vi "Aux TE Controllers Runtime (2).vi"(8 "Error In":errorcluster, 9 "TE Serial Ports In":T4[](array[typedef]) {"XOFF Char" format="%.0x"; "XON Char" format="%.0x"; "flow control" items=["None"=0, "XON/XOFF"=1, "RTS/CTS"=2, "DTR/DSR"=4]; "stop bits" items=["1.0"=10, "1.5"=15, "2.0"=20]; "data bits" min=5 max=8 step=1; "baud rate" items=["75"=75, "110"=110, "134"=134, "150"=150, "300"=300, "600"=600, "1200"=1200, "1800"=1800, "2400"=2400, "4800"=4800, "7200"=7200, "9600"=9600, "14400"=14400, "19200"=19200, "28800"=28800, "38400"=38400, "56000"=56000, "57600"=57600, "115200"=115200, "128000"=128000, "230400"=230400]; "termination char" format="%.0x"}, 10 "CmdsToWrite":string[](array[string]), 11 "Refs":T1 {"Current Settings"."Pump" items=["Pump 0", "Pump 1", "Pump 2", "Pump 3", "Pump 4", "Pump 5"]; "Current Settings"."Chart X axis Timescale" min=20 max=180 step=1; "Current Settings"."RunTime Mode Settings"."Exp. Gas Tank" items=["0.07", "0.031", "0.877", "1.863", "3.881", "5.790", "7.688", "6.000"]; "Current Settings"."RunTime Mode Settings"."Insp. Gas Tank" items=["0.07", "0.031", "0.877", "1.863", "3.881", "5.790", "7.688", "6.000"]; "Current Settings"."RunTime Mode Settings"."I:E Ratio" max=30 scale=0.0..7.0; "Current Settings"."RunTime Mode Settings"."Resp Rate Brpm" min=0 max=30 format="%.2f"; "Current Settings"."TE#2 Configuration"."Serial Port"."XOFF Char" format="%.0x"; "Current Settings"."TE#2 Configuration"."Serial Port"."XON Char" format="%.0x"; "Current Settings"."TE#2 Configuration"."Serial Port"."flow control" items=["None"=0, "XON/XOFF"=1, "RTS/CTS"=2, "DTR/DSR"=4]; "Current Settings"."TE#2 Configuration"."Serial Port"."stop bits" items=["1.0"=10, "1.5"=15, "2.0"=20]; "Current Settings"."TE#2 Configuration"."Serial Port"."data bits" min=5 max=8 step=1; "Current Settings"."TE#2 Configuration"."Serial Port"."baud rate" items=["75"=75, "110"=110, "134"=134, "150"=150, "300"=300, "600"=600, "1200"=1200, "1800"=1800, "2400"=2400, "4800"=4800, "7200"=7200, "9600"=9600, "14400"=14400, "19200"=19200, "28800"=28800, "38400"=38400, "56000"=56000, "57600"=57600, "115200"=115200, "128000"=128000, "230400"=230400]; "Current Settings"."TE#2 Configuration"."Serial Port"."termination char" format="%.0x"; "Current Settings"."TE#1 Configuration"."Serial Port"."XOFF Char" format="%.0x"; "Current Settings"."TE#1 Configuration"."Serial Port"."XON Char" format="%.0x"; "Current Settings"."TE#1 Configuration"."Serial Port"."flow control" items=["None"=0, "XON/XOFF"=1, "RTS/CTS"=2, "DTR/DSR"=4]; "Current Settings"."TE#1 Configuration"."Serial Port"."stop bits" items=["1.0"=10, "1.5"=15, "2.0"=20]; "Current Settings"."TE#1 Configuration"."Serial Port"."data bits" min=5 max=8 step=1; "Current Settings"."TE#1 Configuration"."Serial Port"."baud rate" items=["75"=75, "110"=110, "134"=134, "150"=150, "300"=300, "600"=600, "1200"=1200, "1800"=1800, "2400"=2400, "4800"=4800, "7200"=7200, "9600"=9600, "14400"=14400, "19200"=19200, "28800"=28800, "38400"=38400, "56000"=56000, "57600"=57600, "115200"=115200, "128000"=128000, "230400"=230400]; "Current Settings"."TE#1 Configuration"."Serial Port"."termination char" format="%.0x"; "Current Settings"."Capnometer Configuration"."Device" items=["None", "TidalWave", "LoFlow / Canary", "Capnogard"]; "Current Settings"."Capnometer Configuration"."Serial Port"."XOFF Char" format="%.0x"; "Current Settings"."Capnometer Configuration"."Serial Port"."XON Char" format="%.0x"; "Current Settings"."Capnometer Configuration"."Serial Port"."flow control" items=["None"=0, "XON/XOFF"=1, "RTS/CTS"=2, "DTR/DSR"=4]; "Current Settings"."Capnometer Configuration"."Serial Port"."stop bits" items=["1.0"=10, "1.5"=15, "2.0"=20]; "Current Settings"."Capnometer Configuration"."Serial Port"."data bits" min=5 max=8 step=1; "Current Settings"."Capnometer Configuration"."Serial Port"."baud rate" items=["75"=75, "110"=110, "134"=134, "150"=150, "300"=300, "600"=600, "1200"=1200, "1800"=1800, "2400"=2400, "4800"=4800, "7200"=7200, "9600"=9600, "14400"=14400, "19200"=19200, "28800"=28800, "38400"=38400, "56000"=56000, "57600"=57600, "115200"=115200, "128000"=128000, "230400"=230400]; "Current Settings"."Capnometer Configuration"."Serial Port"."termination char" format="%.0x"; "Current Settings"."DAQx Settings"."Analog Output Settings (Volts)" format="%#.3g"; "Current Settings"."DAQx Settings"."Duty Cycle" min=10.0 max=90.0 format="%.1g"; "Current Settings"."DAQx Settings"."Frequency" min=20.0 max=200.0; "Current Settings"."DataLogging Settings"."Data File Duration (Minutes)" min=2 max=200 format="%#.2g"; "Current Settings"."Calibration Settings"."Tolerance #2" min=2 max=4096; "Current Settings"."Calibration Settings"."Cal. Average" min=2 max=4096; "Current Settings"."Test Settings"."Test Sensor ID" items=["(select)", "RB", "YC", "", "Other"]}) -> (0 "Error Out":errorcluster, 1 "Read Array":string[][](array[string]), 2 "ReadData":sgl[][](array[numeric]) format="%.2g", 3 "TE Serial Ports Out":T4[](array[typedef]) {"XOFF Char" format="%.0x"; "XON Char" format="%.0x"; "flow control" items=["None"=0, "XON/XOFF"=1, "RTS/CTS"=2, "DTR/DSR"=4]; "stop bits" items=["1.0"=10, "1.5"=15, "2.0"=20]; "data bits" min=5 max=8 step=1; "baud rate" items=["75"=75, "110"=110, "134"=134, "150"=150, "300"=300, "600"=600, "1200"=1200, "1800"=1800, "2400"=2400, "4800"=4800, "7200"=7200, "9600"=9600, "14400"=14400, "19200"=19200, "28800"=28800, "38400"=38400, "56000"=56000, "57600"=57600, "115200"=115200, "128000"=128000, "230400"=230400]; "termination char" format="%.0x"}, 4 "TE Bytes Read":i16[][](array[numeric]), 5 "Set Point Good":bool, 6 "TE Data":sgl[][](array[numeric]), 7 "Set Point Disabled":bool)   [LabVIEW 2015]
uses:
  Controls/Serial Visa Control.ctl
  Controls/DAQ Needed.ctl
  Controls/Processed Variables.ctl
  Controls/AirPump Controls.ctl
  Controls/IE Ratio knob.ctl
  Controls/UI Settings.ctl
  Controls/Aux CO2 Control.ctl
  Controls/Aux CO2 Selector.ctl
  Controls/Aux TE Control.ctl
  Controls/Queues And Others.ctl
  Controls/SerialPortControl.ctl
  Miscellaneous/Globals.vi
panel:
  out "after substring":string
  out "appended array":string[][](array[string])
  out "subarray":dbl[](array[numeric])
  out "size(s)":i32[](array[numeric])
  # "Note: Setting Brpm to zero will\ndisable Insp / Exp digital output."
  # "mmHg"
  # "pts"
  # "tolerance"
  # "AN5 (Temp 1)"
  # "AN6 (Temp 2)"
  # "AN7 (Temp 3)"
  # "AN8 (T FET)"
  # "AN0 (T POT)"
  # "Tref (Set Pt))"
  # "(Spare)"
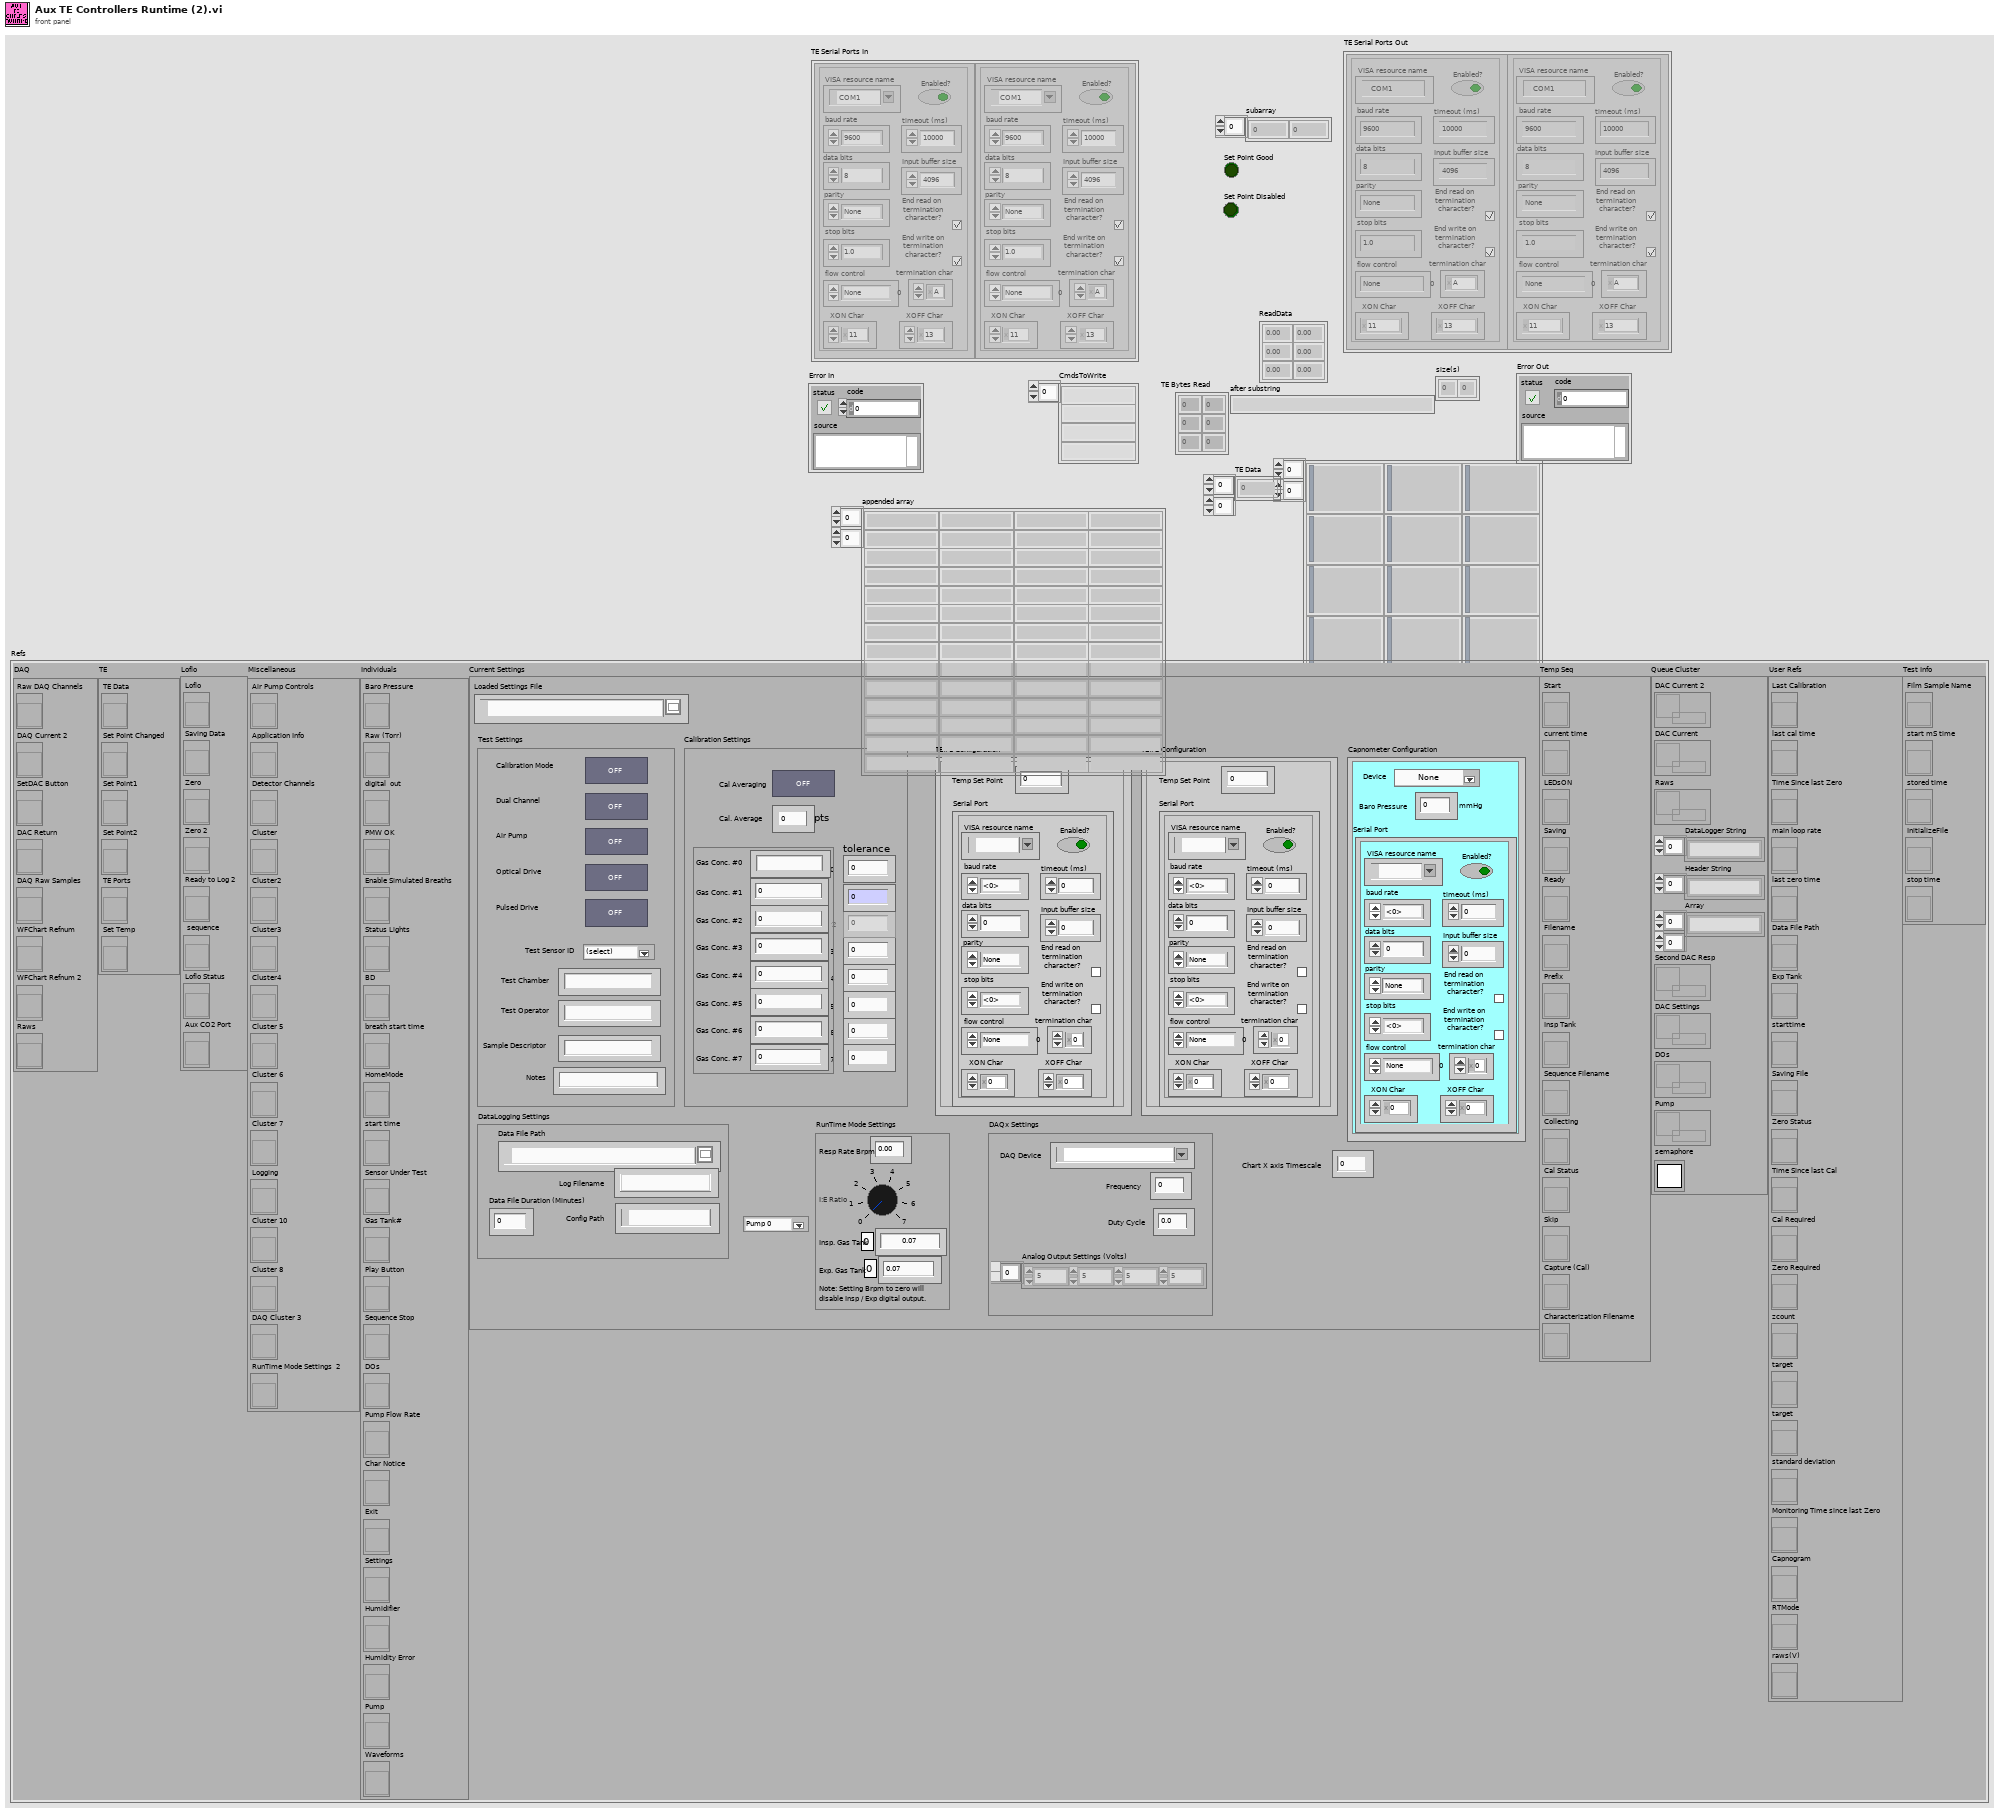
[diagram p1: front panel]
types:
  T1 = typedef "DAQ Needed.ctl" = cluster{"DAQ":cluster{"Raw DAQ Channels":refnum<vi>, "DAQ Current 2":refnum<vi>, "SetDAC Button":refnum<vi>, "DAC Return":refnum<vi>, "DAQ Raw Samples":refnum<vi>, "WFChart Refnum":refnum<vi>, "WFChart Refnum 2":refnum<vi>, "Raws":refnum<vi>}, "TE":cluster{"TE Data":refnum<vi>, "Set Point Changed":refnum<vi>, "Set Point1":refnum<vi>, "Set Point2":refnum<vi>, "TE Ports":refnum<vi>, "Set Temp":refnum<vi>}, "Loflo":cluster{"Loflo":refnum<vi>, "Saving Data":refnum<vi>, "Zero":refnum<vi>, "Zero 2":refnum<vi>, "Ready to Log 2":refnum<vi>, " sequence":refnum<vi>, "Loflo Status ":refnum<vi>, "Aux CO2 Port":refnum<vi>}, "Miscellaneous":cluster{"Air Pump Controls":refnum<vi>, "Application Info":refnum<vi>, "Detector Channels ":refnum<vi>, "Cluster":refnum<vi>, "Cluster2":refnum<vi>, "Cluster3":refnum<vi>, "Cluster4":refnum<vi>, "Cluster 5":refnum<vi>, "Cluster 6":refnum<vi>, "Cluster 7":refnum<vi>, "Logging":refnum<vi>, "Cluster 10":refnum<vi>, "Cluster 8":refnum<vi>, "DAQ Cluster 3":refnum<vi>, "RunTime Mode Settings  2":refnum<vi>}, "Individuals":cluster{"Baro Pressure":refnum<vi>, "Raw (Torr)":refnum<vi>, "digital  out":refnum<vi>, "PMW OK":refnum<vi>, "Enable Simulated Breaths":refnum<vi>, "Status Lights":refnum<vi>, "BD":refnum<vi>, "breath start time":refnum<vi>, "HomeMode":refnum<vi>, "start time":refnum<vi>, "Sensor Under Test":refnum<vi>, "Gas Tank#":refnum<vi>, "Play Button":refnum<vi>, "Sequence Stop":refnum<vi>, "DOs":refnum<vi>, "Pump Flow Rate":refnum<vi>, "Char Notice":refnum<vi>, "Exit":refnum<vi>, "Settings":refnum<vi>, "Humidifier":refnum<vi>, "Humidity Error":refnum<vi>, "Pump":refnum<vi>, "Waveforms":refnum<vi>}, "Current Settings":T2, "Temp Seq":cluster{"Start":refnum<vi>, "current time":refnum<vi>, "LEDsON":refnum<vi>, "Saving":refnum<vi>, "Ready":refnum<vi>, "Filename":refnum<vi>, "Prefix":refnum<vi>, "Insp Tank":refnum<vi>, "Sequence Filename":refnum<vi>, "Collecting":refnum<vi>, "Cal Status":refnum<vi>, "Skip":refnum<vi>, "Capture (Cal)":refnum<vi>, "Characterization Filename":refnum<vi>}, "Queue Cluster":T7, "User Refs":cluster{"Last Calibration":refnum<vi>, "last cal time":refnum<vi>, "Time Since last Zero":refnum<vi>, "main loop rate":refnum<vi>, "last zero time":refnum<vi>, "Data File Path":refnum<vi>, "Exp Tank":refnum<vi>, "starttime":refnum<vi>, "Saving File":refnum<vi>, "Zero Status":refnum<vi>, "Time Since last Cal":refnum<vi>, "Cal Required":refnum<vi>, "Zero Required":refnum<vi>, "zcount":refnum<vi>, "target":refnum<vi>, "target":refnum<vi>, "standard deviation":refnum<vi>, "Monitoring Time since last Zero":refnum<vi>, "Capnogram":refnum<vi>, "RTMode":refnum<vi>, "raws(V)":refnum<vi>}, "Test Info":cluster{"Film Sample Name":refnum<vi>, "start mS time":refnum<vi>, "stored time":refnum<vi>, "InitializeFile":refnum<vi>, "stop time":refnum<vi>}}
  T2 = typedef "UI Settings.ctl" = cluster{"Loaded Settings File":path, "Test Settings":cluster{"Dual Channel":bool, "Air Pump":bool, "Optical Drive":bool, "Pulsed Drive":bool, "Calibration Mode":bool, "Test Sensor ID":u16, "Test Chamber":string, "Test Operator":string, "Sample Descriptor":string, "Notes":string}, "Calibration Settings":cluster{"Cal. Average":u16, "Cal Averaging":bool, "Tolerance #0":sgl, "Tolerance #7":sgl, "Tolerance #6":sgl, "Tolerance #5":sgl, "Tolerance #4":sgl, "Tolerance #3":sgl, "Tolerance #2":sgl, "Tolerance #1":sgl, "Gas Tank Settings":cluster{"Gas Conc. #0":string, "Gas Conc. #1":sgl, "Gas Conc. #2":sgl, "Gas Conc. #3":sgl, "Gas Conc. #4":sgl, "Gas Conc. #5":sgl, "Gas Conc. #6":sgl, "Gas Conc. #7":sgl}}, "DataLogging Settings":cluster{"Data File Path":path, "Data File Duration (Minutes)":sgl, "Log Filename":string, "Config Path":path}, "DAQx Settings":cluster{"DAQ Device":tag, "Frequency":dbl, "Duty Cycle":dbl, "Analog Output Settings (Volts)":sgl[]}, "Capnometer Configuration":T3, "TE#1 Configuration":T6, "TE#2 Configuration":T6, "RunTime Mode Settings ":cluster{"Resp Rate Brpm ":sgl, "I:E Ratio":u8, "Insp. Gas Tank":u16, "Exp. Gas Tank":u16}, "Chart X axis Timescale":u16, "Pump":u16}
  T3 = typedef "Aux CO2 Control.ctl" = cluster{"Serial Port":T4, "Baro Pressure":u32, "Device":T5}
  T4 = typedef "Serial Visa Control.ctl" = cluster{"termination char":u8, "End read on termination character?":bool, "Enabled?":bool, "VISA resource name":refnum<visa-resource-name>, "baud rate":u32, "data bits":u16, "parity":enum16{"None", "Odd", "Even", "Mark", "Space"}, "stop bits":u16, "flow control":u16, "timeout (ms)":u32, "Input buffer size":u32, "End write on termination character?":bool, "XON Char":u8, "XOFF Char":u8}
  T5 = typedef "Aux CO2 Selector.ctl" = u16
  T6 = typedef "Aux TE Control.ctl" = cluster{"Temp Set Point":sgl, "Serial Port":T4}
  T7 = typedef "Queues And Others.ctl" = cluster{"DAC Current 2":refnum<queue>, "DAC Current":refnum<queue>, "Raws":refnum<queue>, "DataLogger String":string[], "Header String":string[], "Array":string[][], "Second DAC Resp":refnum<queue>, "DAC Settings":refnum<queue>, "DOs":refnum<queue>, "Pump":refnum<queue>, "semaphore":T8}
  T8 = typedef "Semaphore RefNum" = refnum<k1>
  T9 = typedef "SerialPortControl.ctl" = enum16{"Initialize", "Write Data", "Read Data", "Close Port"}
  T10 = cluster{"Ref CO2":sgl, "Humidity":sgl, "TE #1":sgl, "TE #2":sgl, " Film `C":dbl, "Bath `C":dbl, " Det. `C":dbl, " Ambient":dbl, " Chamber C ":dbl}
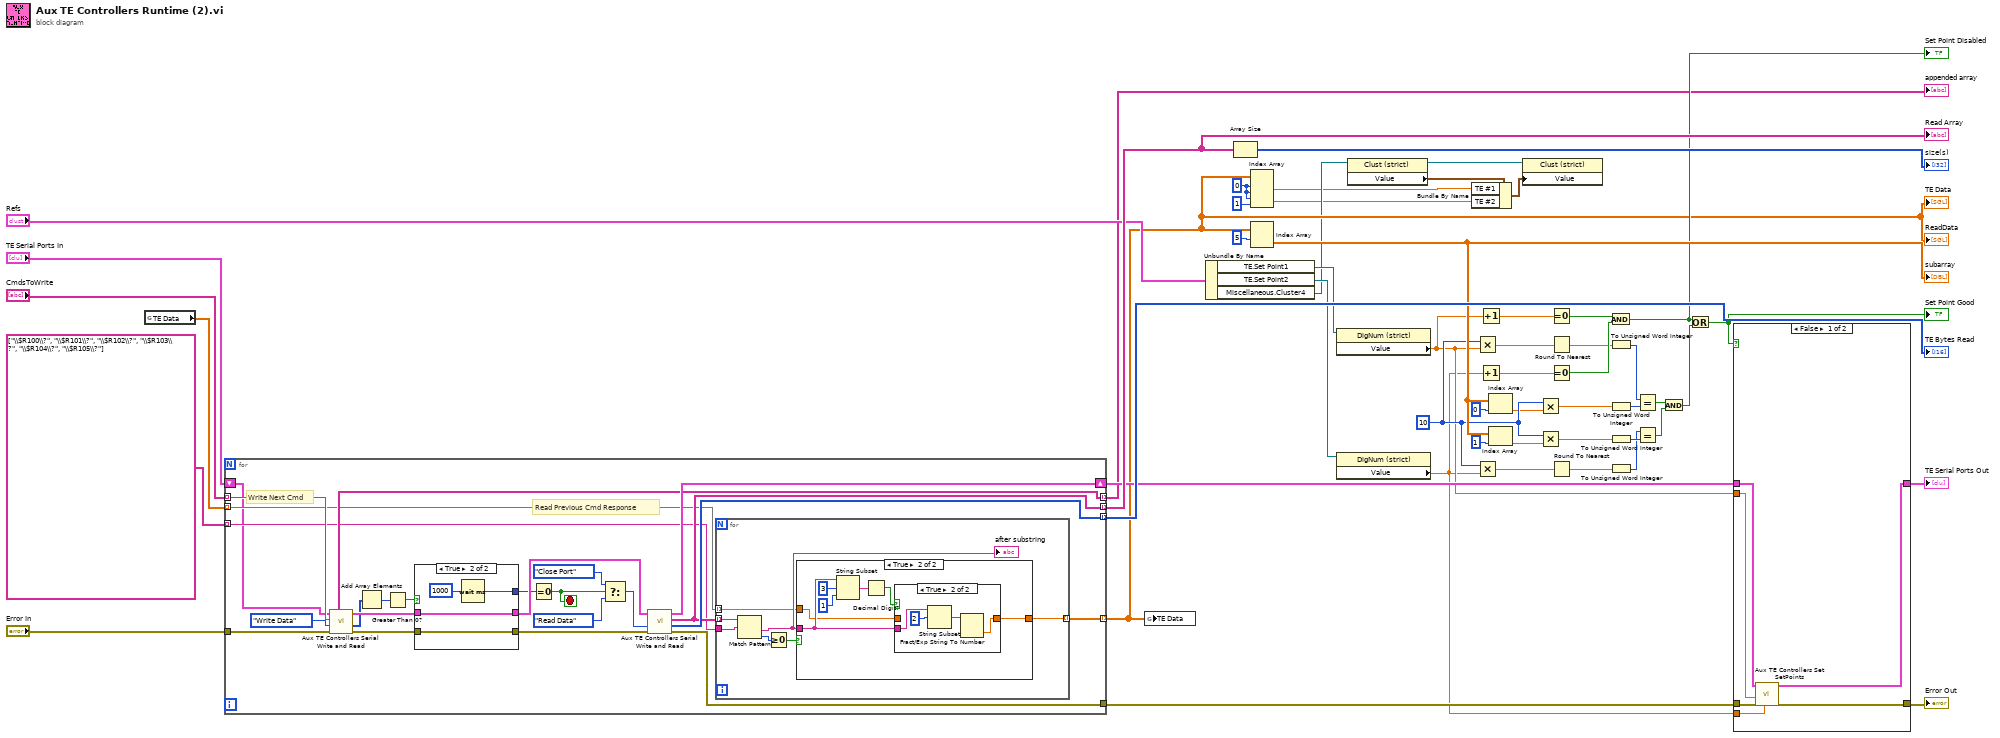
[diagram p0: block diagram]
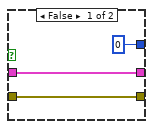
[diagram p5: hidden frame]
diagram:
  w16 = 0 ("index (row)")
  w40 = 10
  n1 = global read "Globals.vi" "TE Data"() -> (w10:sgl[][])
  n2 = for {
    tunnel: [w74] -> w33
    tunnel: "Error In" -> [w76]
    tunnel: [w73] -> w51 mode=indexing
    tunnel: "CmdsToWrite" -> [w58] mode=indexing
    tunnel: [w59] -> w52 mode=indexing
    tunnel: [w57] -> w9 mode=indexing
    tunnel: [w60] -> w11 mode=indexing
    tunnel: string[] ["\\$R100\\?", "\\$R101\\?", "\\$R102\\?", "\\$R103\\?", "\\$R104\\?", "\\$R105\\?"] ("CmdsToWrite") -> [w56] mode=indexing
    tunnel: w10 -> [w55] mode=indexing
    shift-right: [w75] -> w35
    shift-left: "TE Serial Ports In" -> [w54]
    stop <- w61 stop-if-true
    # "Read Previous Cmd Response"
    # "Write Next Cmd"
    n3 = call "Aux TE Controllers Serial Write and Read.vi"("error in"=w76, "Action"=SerialPortControl."Write Data", "string to write"=w58, "TE Controller Serial Ports In"=w54) -> ("Error Out"=w70:errorcluster, "#Bytes R/W"=w66:i16[], "TE Controller Serial Ports Out"=w72:T4[], "appended array"=w60:string[])  [unwired: 1 in, 1 out]
    n4 = Add Array Elements(numeric array=w66) -> (sum=w68:i16)
    n5 = Greater Than 0?(x=w68) -> (x > 0?=w67:bool)
    n6 = case shown="True" w67 {
      tunnel: [w99 w104] -> w71
      tunnel: w72 -> [w99 w104]
      tunnel: [w100 w103] -> w69
      tunnel: w70 -> [w100 w103]
      tunnel: [u32 0 ("millisecond timer value") w101] -> w65
      frame False {
      }
      frame True {
        n7 = Wait (ms)(milliseconds to wait=i16 1000 ("y")) -> (millisecond timer value=w101:u32)
      }
    }
    n8 = Equal To 0?(x=w65) -> (x = 0?=w61:bool)
    n9 = Select(t=SerialPortControl."Close Port" ("Action"), s=w61, f=SerialPortControl."Read Data" ("Action")) -> (s? t:f=w64:T9)
    n10 = call "Aux TE Controllers Serial Write and Read.vi"("error in"=w69, "Action"=w64, "TE Controller Serial Ports In"=w71) -> ("Error Out"=w74:errorcluster, "#Bytes R/W"=w73:i16[], "Data Read"=w59:string[], "TE Controller Serial Ports Out"=w75:T4[])  [unwired: 2 in, 1 out]
    n11 = for {
      tunnel: w59 -> [w84] mode=indexing
      tunnel: w56 -> [w83]
      tunnel: [w81] -> w57 mode=indexing
      tunnel: w55 -> [w80] mode=indexing
      n12 = Match Pattern(string=w84, regular expression=w83) -> (after substring=w82:string, offset past match=w79:i32)  [unwired: 1 in, 2 out]
      "after substring" <- w82
      n13 = Greater Or Equal To 0?(x=w79) -> (x >= 0?=w78:bool)
      n14 = case shown="True" w78 {
        tunnel: w82 -> [_ w87]
        tunnel: [w85 w92] -> w81
        tunnel: w80 -> [w85 w86]
        frame False {
        }
        frame True {
          n15 = String Subset(string=w87, offset (0)=3, length (rest)=1 ("length (rest)")) -> (substring=w89:string)
          n16 = Decimal Digit?(1:w89) -> (0:w88:bool)
          n17 = case shown="True" w88 {
            tunnel: [w93 w97] -> w92
            tunnel: w87 -> [_ w95]
            tunnel: w86 -> [w93 _]
            frame False {
            }
            frame True {
              n18 = String Subset(string=w95, offset (0)=2) -> (substring=w94:string)  [unwired: 1 in]
              n19 = Fract/Exp String To Number(string=w94) -> (number=w97:dbl)  [unwired: 3 in, 1 out]
            }
          }
        }
      }
    }
  }
  "TE Bytes Read" <- w51
  "Read Array" <- w52
  "ReadData" <- w9
  "TE Data" <- w9
  "appended array" <- w11
  n20 = global write "Globals.vi" "TE Data"(w9) -> ()
  n21 = Unbundle By Name("Refs") -> ("TE.Set Point1"=w13:refnum<vi>, "TE.Set Point2"=w12:refnum<vi>, "Miscellaneous.Cluster4"=w6:refnum<vi>)
  n22 = Array Size(array=w52) -> (size(s)=→"size(s)":i32[])
  n23 = Index Array(array=w9, index (row) #1=w16, index (col) #1=w16, index (row) #2=w16, index (col) #2=1 ("disabled index (col)")) -> (element #1=w2:dbl, element #2=w1:dbl)
  n24 = Index Array(array=w9, index (row)=5) -> (element=w45:dbl[])  [unwired: 1 in]
  "subarray" <- w45
  n25 = property class="DigNum (strict)"(reference=w13) -> ("Value"=w18:sgl)  [unwired: 1 in, 2 out]
  n26 = property class="DigNum (strict)"(reference=w12) -> ("Value"=w17:sgl)  [unwired: 1 in, 2 out]
  n27 = property class="Clust (strict)"(reference=w6) -> (reference out=w5:refnum<vi>, "Value"=w4:T10)  [unwired: 1 in, 1 out]
  n28 = Bundle By Name(cluster=w4, "TE #1"=w2, "TE #2"=w1) -> (w3:T10)
  n29 = Multiply(x=w40, y=w18) -> (x*y=w21:sgl)
  n30 = Multiply(x=w40, y=w17) -> (x*y=w23:sgl)
  n31 = Increment(x=w18) -> (x+1=w31:sgl)
  n32 = Increment(x=w17) -> (x+1=w30:sgl)
  n33 = Index Array(array=w45, index=0) -> (element=w39:dbl)
  n34 = Index Array(array=w45, index=1) -> (element=w41:dbl)
  n35 = property class="Clust (strict)"(reference=w5, "Value"=w3) -> ()  [unwired: 1 in, 2 out]
  n36 = Multiply(x=w40, y=w39) -> (x*y=w22:dbl)
  n37 = Multiply(x=w40, y=w41) -> (x*y=w24:dbl)
  n38 = Equal To 0?(x=w31) -> (x = 0?=w28:bool)
  n39 = Round To Nearest(number=w21) -> (nearest integer value=w20:sgl)
  n40 = Equal To 0?(x=w30) -> (x = 0?=w29:bool)
  n41 = Round To Nearest(number=w23) -> (nearest integer value=w19:sgl)
  n42 = And(x=w28, y=w29) -> (x .and. y?=w25:bool)
  "Set Point Disabled" <- w25
  n43 = To Unsigned Word Integer(number=w20) -> (unsigned 16bit integer=w36:u16)
  n44 = To Unsigned Word Integer(number=w22) -> (unsigned 16bit integer=w37:u16)
  n45 = To Unsigned Word Integer(number=w24) -> (unsigned 16bit integer=w42:u16)
  n46 = To Unsigned Word Integer(number=w19) -> (unsigned 16bit integer=w38:u16)
  n47 = Equal?(x=w36, y=w37) -> (x = y?=w43:bool)
  n48 = Equal?(x=w38, y=w42) -> (x = y?=w44:bool)
  n49 = And(x=w43, y=w44) -> (x .and. y?=w27:bool)
  n50 = Or(x=w25, y=w27) -> (x .or. y?=w26:bool)
  "Set Point Good" <- w26
  n51 = case shown="False" w26 {
    tunnel: [w107 w112] -> w34
    tunnel: w35 -> [w110 w112]
    tunnel: [w108 w111] -> w32
    tunnel: w33 -> [w109 w111]
    tunnel: w18 -> [w106 _]
    tunnel: w17 -> [w105 _]
    frame False {
      n52 = call "Aux TE Controllers Set SetPoints.vi"("Set Point2"=w105, "Error In"=w109, "Set Point1"=w106, "TE Serial Ports In"=w110) -> ("Error Out"=w108:errorcluster, "TE Serial Ports Out"=w107:T4[])  [unwired: 5 in, 1 out]
    }
    frame True {
    }
  }
  "TE Serial Ports Out" <- w34
  "Error Out" <- w32
